vi "tcp 읽기2.vi"() -> ()   [LabVIEW 2014]
uses:
  <vilib>/Utility/sysdir.llb/System Directory Type.ctl
panel:
  out "결과":string
  out "원소":i16
  out "뒤집힌 배열 2":i16[](array[numeric])
  out "key의숫자값":i16[](array[numeric])
  in  "stop 2":bool
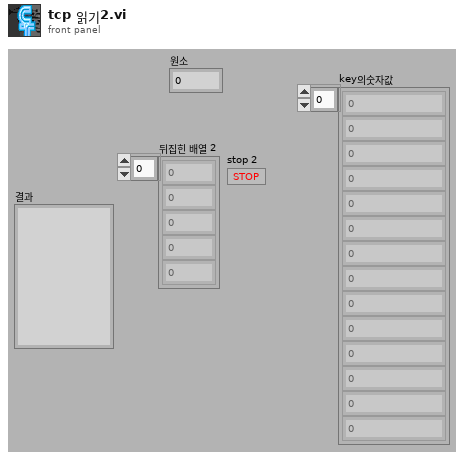
[diagram p1: front panel]
types:
  T1 = enum16{"open", "replace", "create", "open or create", "replace or create", "replace or create with confirmation"}
  T2 = typedef "System Directory Type.ctl" = i32
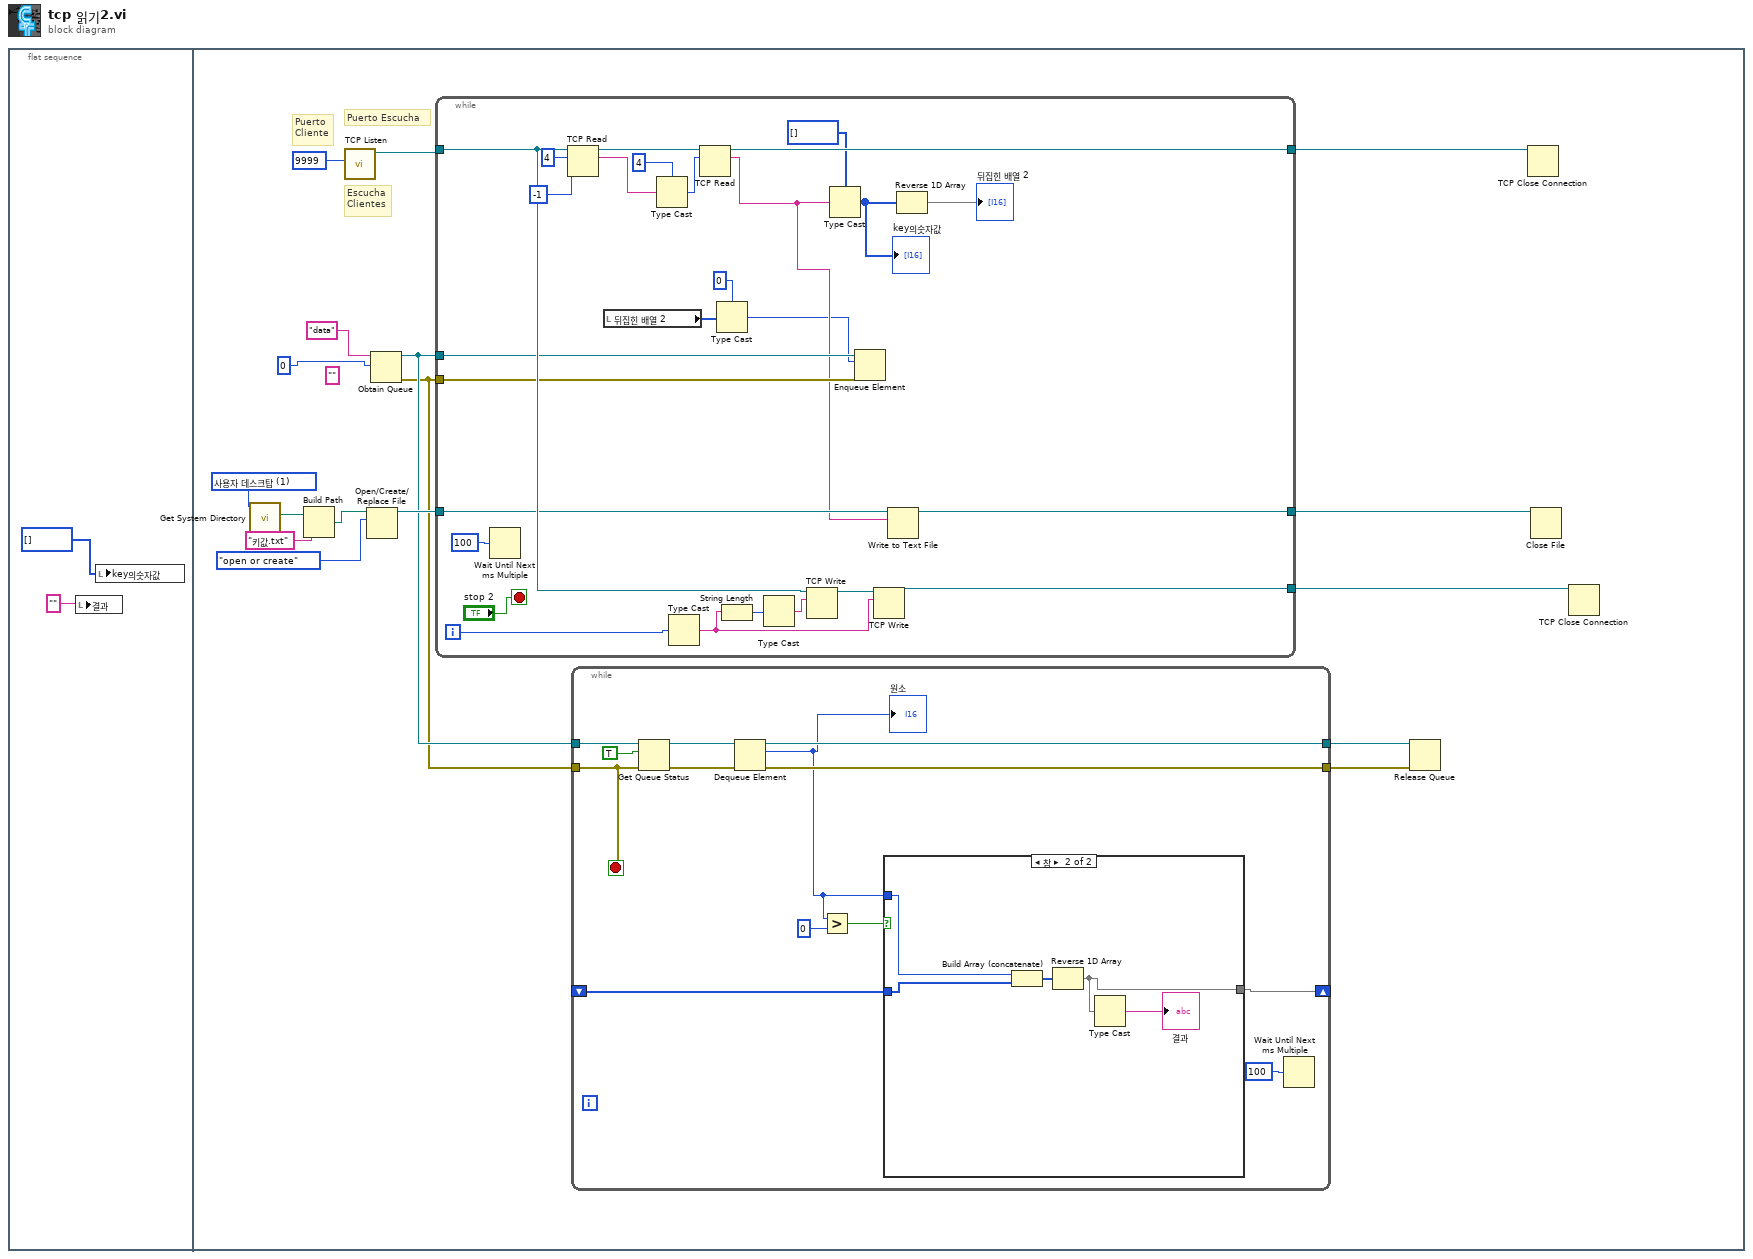
[diagram p0: block diagram]
diagram:
  n1 = flat-sequence {
    frame #0 {
      n2 = local write "결과"("") -> ()
      n3 = local write "key의숫자값"(i16[] []) -> ()
    }
    frame #1 {
      (unwired) ""
      w14 = T2 1 items=["사용자 홈"=0, "사용자 데스크탑"=1, "사용자 문서"=2, "사용자 어플리케이션 데이터"=3, "사용자 환경"=4, "사용자 임시"=5, "퍼블릭 문서"=6, "퍼블릭 어플리케이션 데이터"=7, "퍼블릭 환경"=8, "퍼블릭 캐시"=13, "시스템 코어 라이브러리"=9, "시스템 설치된 라이브러리"=10, "어플리케이션 파일"=11, "부팅 볼륨 루트"=12] ("system directory type")
      # "Puerto\nCliente"
      # "Escucha\nClientes"
      # "Puerto Escucha"
      n4 = call <vilib>:"Get System Directory.vi"("system directory type"=w14) -> ("system directory"=w13:path)  [unwired: 10 in]
      n5 = Build Path(base path=w13, name or relative path="키값.txt" ("이름 또는 상대 경로")) -> (appended path=w10:path)
      n6 = call <vilib>:"TCP Listen.vi"("port"=u16 9999) -> ("connection ID"=w17:refnum<k5>)  [unwired: 6 in, 4 out]
      n7 = Open/Create/Replace File(file path (use dialog)=w10, operation (0:open)=T1."open or create" ("동작(0:open)")) -> (refnum out=w9:refnum<file>)  [unwired: 4 in, 2 out]
      n8 = Obtain Queue(name (unnamed)="data" ("이름(이름없음)"), element data type=i16 0) -> (queue out=w7:refnum<queue>, error out=w4:errorcluster)  [unwired: 3 in, 1 out]
      n9 = while {
        tunnel: w17 -> [w55]
        tunnel: [w64] -> w18
        tunnel: [w57] -> w16
        tunnel: w9 -> [w48]
        tunnel: [w49] -> w15
        tunnel: w7 -> [w47]
        tunnel: w4 -> [w46]
        i -> [w56]
        stop <- "stop 2" stop-if-true
        n10 = Wait Until Next ms Multiple(millisecond multiple=u32 100) -> ()  [unwired: 1 out]
        n11 = TCP Read(connection ID=w55, bytes to read=4, 9:-1 ("타임아웃 ms (25000)")) -> (connection ID out=w52:refnum<k5>, data out=w54:string)  [unwired: 2 in, 1 out]
        n12 = local read "뒤집힌 배열 2"() -> (w43:i16[])
        n13 = Type Cast(type=4 ("bytes to read"), x=w54) -> (*(type *) &x=w44:i32)
        n14 = Type Cast(x=w56) -> (*(type *) &x=w58:string)  [unwired: 1 in]
        n15 = TCP Read(connection ID=w52, bytes to read=w44) -> (connection ID out=w64:refnum<k5>, data out=w45:string)  [unwired: 3 in, 1 out]
        n16 = Type Cast(type=i16 0, x=w43) -> (*(type *) &x=w41:i16)
        n17 = String Length(string=w58) -> (length=w59:i32)
        n18 = Type Cast(x=w59) -> (*(type *) &x=w60:string)  [unwired: 1 in]
        n19 = TCP Write(connection ID=w55, data in=w60) -> (connection ID out=w61:refnum<k5>)  [unwired: 2 in, 2 out]
        n20 = Type Cast(type=i16[] [], x=w45) -> (*(type *) &x=w39:i16[])
        "key의숫자값" <- w39
        n21 = Enqueue Element(queue=w47, element=w41, error in (no error)=w46) -> ()  [unwired: 1 in, 3 out]
        n22 = TCP Write(connection ID=w61, data in=w58) -> (connection ID out=w57:refnum<k5>)  [unwired: 2 in, 2 out]
        n23 = Write to Text File(file (use dialog)=w48, text=w45) -> (refnum out=w49:refnum<file>)  [unwired: 2 in, 2 out]
        n24 = Reverse 1D Array(array=w39) -> (reversed array=→"뒤집힌 배열 2":i16[])
      }
      n25 = while {
        tunnel: w4 -> [w26]
        tunnel: w7 -> [w32]
        tunnel: [w29] -> w6
        tunnel: [w28] -> w5
        shift-right: [w21] -> _
        shift-left: _ -> [w22]
        stop <- w26 stop-if-true
        n26 = Get Queue Status(queue=w32, return elements? (F)=TRUE ("원소 반환? (거짓)"), error in (no error)=w26) -> (queue out=w30:refnum<queue>, error out=w31:errorcluster)  [unwired: 6 out]
        n27 = Dequeue Element(queue=w30, error in (no error)=w31) -> (queue out=w29:refnum<queue>, element=w20:i16, error out=w28:errorcluster)  [unwired: 1 in, 1 out]
        "원소" <- w20
        n28 = Greater?(x=w20, y=i16 0) -> (0:w23:bool)
        n29 = case shown="참" w23 {
          tunnel: w22 -> [w33 w38]
          tunnel: w20 -> [_ w37]
          tunnel: [w33 w35] -> w21
          frame False {
          }
          frame True {
            n30 = Build Array (concatenate)(w37, w38) -> (w36:i16[])
            n31 = Reverse 1D Array(array=w36) -> (reversed array=w35:i16[])
            n32 = Type Cast(x=w35) -> (*(type *) &x=→"결과":string)  [unwired: 1 in]
          }
        }
        n33 = Wait Until Next ms Multiple(millisecond multiple=u32 100) -> ()  [unwired: 1 out]
      }
      n34 = Release Queue(queue=w6, error in (no error)=w5) -> ()  [unwired: 1 in, 3 out]
      n35 = TCP Close Connection(connection ID=w18) -> ()  [unwired: 2 in, 2 out]
      n36 = Close File(refnum=w15) -> ()  [unwired: 1 in, 2 out]
      n37 = TCP Close Connection(connection ID=w16) -> ()  [unwired: 2 in, 2 out]
    }
  }
